vi "LessThanOffset.vi"(1 "offset":i32=1, 2 "Position":i32, 3 "Numeric":i32) -> (0 "Boolean":bool)   [LabVIEW 2014]
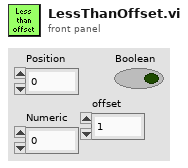
[diagram p1: front panel]
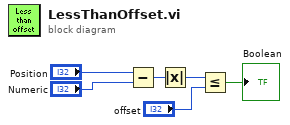
[diagram p0: block diagram]
diagram:
  n1 = Subtract(x="Position", y="Numeric") -> (x-y=w3:i32)
  n2 = Absolute Value(x=w3) -> (abs(x)=w4:i32)
  n3 = Less Or Equal?(x=w4, y="offset") -> (x <= y?=→"Boolean":bool)
